vi "RSZVB Set Pulse Train Segment Start.vi"(7 "Segment Start (0.0 s)":dbl format="%^.3e", 8 "error in (no error)":errorcluster {"code" format="%.0x"}, 9 "Segment (1)":i32=1, 10 "Channel (1)":i32=1, 11 "VISA session":refnum<visa-resource-name>) -> (0 "error out":errorcluster {"code" format="%.0x"}, 3 "dup VISA session":refnum<visa-resource-name>)   [LabVIEW 2011]
doc: "This VI changes the start time of a pulse train segment. A range must be created first to enable this VI (rszvb_DefinePulseTrainSegments). \n\nNote(s):\n\n(1) This VI is available only with option R&S ZVA-K27.\n\nRemote-control command(s):\n[SENSe<Ch>:]PULSe:GENerator<gen_no>:TRAin:SEGMent<Seg>:STARt"
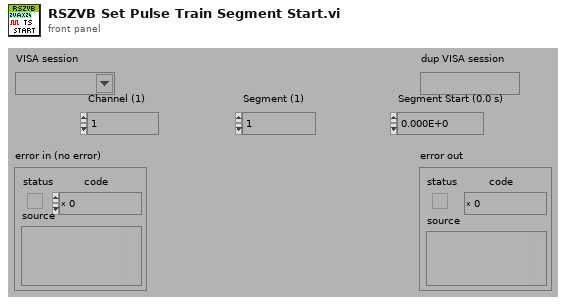
[diagram p1: front panel]
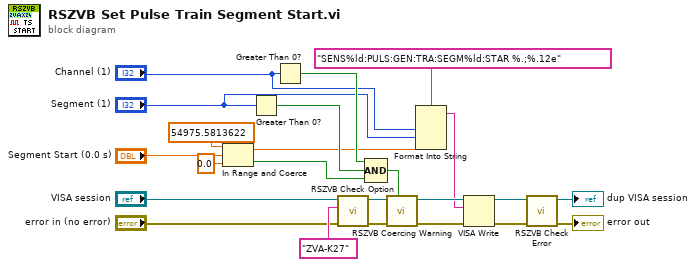
[diagram p0: block diagram]
diagram:
  n1 = In Range and Coerce(upper limit=54975.5813622, x="Segment Start (0.0 s)", lower limit=0.0) -> (coerced(x)=w4:dbl, In Range?=w5:bool)
  n2 = Greater Than 0?(x="Segment (1)") -> (x > 0?=w12:bool)
  n3 = Greater Than 0?(x="Channel (1)") -> (x > 0?=w13:bool)
  n4 = call "RSZVB Check Option.vi"("error in (no error)"="error in (no error)", "Options"="ZVA-K27", "VISA session"="VISA session") -> ("error out"=w17:errorcluster, "dup VISA session"=w16:refnum<visa-resource-name>)  [unwired: 7 in]
  n5 = Compound Arithmetic op=AND(w13, w12, w5) -> (w15:bool)
  n6 = call "RSZVB Coercing Warning.vi"("In Range?"=w15, "error in (no error)"=w17, "VISA session"=w16) -> ("error out"=w22:errorcluster, "dup VISA session"=w23:refnum<visa-resource-name>)  [unwired: 7 in]
  n7 = Format Into String(format string="SENS%ld:PULS:GEN:TRA:SEGM%ld:STAR %.;%.12e", "Channel (1)", "Segment (1)", w4) -> (resulting string=w19:string)  [unwired: 2 in, 1 out]
  n8 = VISA Write(VISA resource name=w23, write buffer=w19, error in (no error)=w22) -> (VISA resource name out=w20:refnum<visa-resource-name>, error out=w21:errorcluster)  [unwired: 1 out]
  n9 = call "RSZVB Check Error.vi"("error in (no error)"=w21, "VISA session"=w20) -> ("error out"=→"error out":errorcluster, "dup VISA session"=→"dup VISA session":refnum<visa-resource-name>)  [unwired: 8 in]
